vi "Grid_Finish_v1.vi"(8 "Error in":errorcluster, 9 "FileRefs":T2, 10 "Settings":T1={"Drift Correction Settings"={"Drift Correction every"=80, "Drift correction Pixels"=256, "Channel index (0-23)"=0, "MaxImagesBack"=2, "Threshold"=2, "Increment"=8, "max applied Drift Correction"=20, "Correct Drift"=TRUE, "Correlate"=0, "Correct z drift"=FALSE, "zdrift \nDuration (s)"=0.0}, "Spectroscopy Setting"={"Imaging Current"=1e-11, "ref Current"=7e-11, "tip Speed (m/s)"=2e-09, "Imaging Bias"=0.02, "ref Bias"=-0.1, "preSTS delay [ms]"=500, "STS z offset"=2e-10, "during Spec Bias (V)"=-0.1, "trigger1 < Hz"=0.0, "trigger 2 >Hz"=0.0, "autoStop"=FALSE, "Spectroscopy"=0, "PLL ON/OFF"=TRUE, "readjust setpoint every "=1, "z Reference"=FALSE, "Lock In"=TRUE}, "Misc"={"File name"="symmetric_node_zOff=200p", "Email when finished"="cornelius.krull@monash.edu,Dhaneesh.Gopalakrishnan@monash.edu,marina.castelli@monash.edu"}, "Grid Settings"={"type"=1, "type order"=1, "X pixel"=0, "Y pixel"=0, "Grid_Parms"={"center X (m)"=0.0, "center Y (m)"=0.0, "width (m)"=0.0, "height (m)"=0.0, "angle (deg)"=0.0}}} {"Grid Settings"."type order" items=["Grid", "Random", "Adam7"]; "Grid Settings"."type" items=["Line", "Grid"]; "Spectroscopy Setting"."Spectroscopy" items=["Bias", "zSpec"]; "Spectroscopy Setting"."trigger 2 >Hz" format="%#_6p"; "Spectroscopy Setting"."trigger1 < Hz" format="%#_6p"; "Spectroscopy Setting"."during Spec Bias (V)" format="%#_5p"; "Spectroscopy Setting"."STS z offset" format="%#_6p"; "Spectroscopy Setting"."ref Bias" format="%#_6p"; "Spectroscopy Setting"."Imaging Bias" format="%#_6p"; "Spectroscopy Setting"."tip Speed (m/s)" format="%.2p"; "Spectroscopy Setting"."ref Current" format="%#_6p"; "Spectroscopy Setting"."Imaging Current" format="%#_6p"; "Drift Correction Settings"."Correlate" items=["first Frame", "successive Frames"]; "Drift Correction Settings"."max applied Drift Correction" min=1 max=100 step=1 format="%.0p"; "Drift Correction Settings"."Threshold" min=1 step=1; "Drift Correction Settings"."Channel index (0-23)" items=["Current"=0, "Z (m)"=14]}, 11 "Application reference":refnum<vi>) -> ()   [LabVIEW 2014]
uses:
  <userlib>/Nanonis Prog Interface V5/Nanonis Prog Interface.lvlib
panel:
  # "z Spectroscopy"
  # "GRID points"
  # "Increase this if no Drift was detected for \na certain number of images"
  # "% of image size"
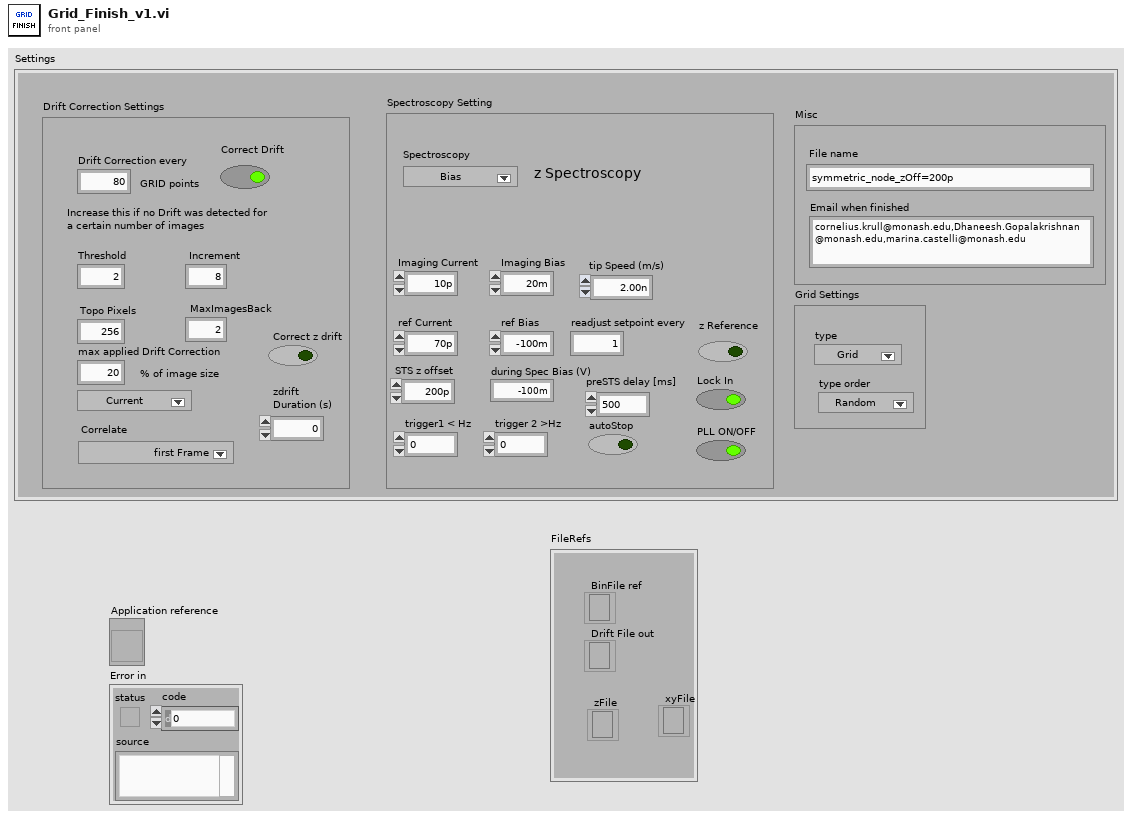
[diagram p1: front panel]
types:
  T1 = cluster{"Drift Correction Settings":cluster{"Drift Correction every":i32, "Drift correction Pixels":i32, "Channel index (0-23)":u8, "MaxImagesBack":i32, "Threshold":i32, "Increment":i32, "max applied Drift Correction":i32, "Correct Drift":bool, "Correlate":u16, "Correct z drift":bool, "zdrift \nDuration (s)":dbl}, "Spectroscopy Setting":cluster{"Imaging Current":dbl, "ref Current":dbl, "tip Speed (m/s)":sgl, "Imaging Bias":dbl, "ref Bias":dbl, "preSTS delay [ms]":u32, "STS z offset":dbl, "during Spec Bias (V)":sgl, "trigger1 < Hz":sgl, "trigger 2 >Hz":sgl, "autoStop":bool, "Spectroscopy":u16, "PLL ON/OFF":bool, "readjust setpoint every ":i32, "z Reference":bool, "Lock In":bool}, "Misc":cluster{"File name":string, "Email when finished":string}, "Grid Settings":cluster{"type":u16, "type order":u16, "X pixel":i32, "Y pixel":i32, "Grid_Parms":cluster{"center X (m)":sgl, "center Y (m)":sgl, "width (m)":sgl, "height (m)":sgl, "angle (deg)":sgl}}}
  T2 = cluster{"Drift File out":refnum<file>, "zFile":refnum<file>, "BinFile ref":refnum<file>, "xyFile":refnum<file>}
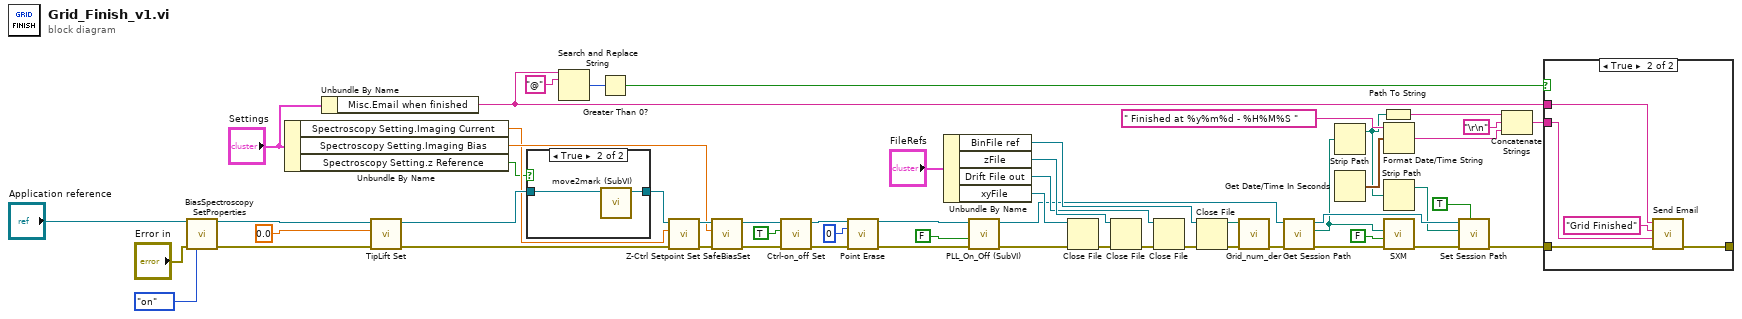
[diagram p0: block diagram]
diagram:
  n1 = call <userlib>:"BiasSpectroscopy SetProperties.vi"("Application ref in"="Application reference", "Error in (no error)"="Error in", "Z-Controller hold (no change)"=enum16{"no change", "on", "off"}."on") -> ("Application ref out"=w45:refnum<vi>, "Error out"=w14:errorcluster)  [unwired: 11 in]
  n2 = Unbundle By Name("Settings") -> ("Spectroscopy Setting.Imaging Current"=w10:dbl, "Spectroscopy Setting.Imaging Bias"=w11:dbl, "Spectroscopy Setting.z Reference"=w1:bool)
  n3 = Unbundle By Name("Settings") -> ("Misc.Email when finished"=w27:string)
  n4 = call <userlib>:"TipLift Set.vi"("error in (no error)"=w14, "TipLift (m)"=sgl 0.0, "Application ref in"=w45) -> ("error out"=w13:errorcluster, "Application ref out"=w42:refnum<vi>)  [unwired: 7 in]
  n5 = case shown="True" w1 {
    tunnel: w42 -> [w57 w59]
    tunnel: [w57 w58] -> w33
    frame False {
    }
    frame True {
      n6 = call "move2mark (SubVI).vi"("Application in"=w59) -> ("Application out"=w58:refnum<vi>)  [unwired: 10 in]
    }
  }
  n7 = Search and Replace String(input string=w27, search string="@") -> (number of replacements=w48:i32)  [unwired: 6 in, 3 out]
  n8 = Greater Than 0?(x=w48) -> (x > 0?=w47:bool)
  n9 = call <userlib>:"Z-Ctrl Setpoint Set.vi"("error in (no error)"=w13, "Z Controller setpoint"=w10, "Application ref in"=w33) -> ("error out"=w12:errorcluster, "Application ref out"=w32:refnum<vi>)  [unwired: 7 in]
  n10 = call "SafeBiasSet.vi"("Application ref in"=w32, "Bias (V)"=w11, "error in (no error)"=w12) -> ("Application ref out"=w39:refnum<vi>, "Error out"=w36:errorcluster)  [unwired: 6 in]
  n11 = call <userlib>:"Ctrl-on_off Set.vi"("error in (no error)"=w36, "Z Controller ON/OFF"=TRUE, "Application ref in"=w39) -> ("error out"=w35:errorcluster, "Application ref out"=w41:refnum<vi>)  [unwired: 7 in]
  n12 = call <userlib>:"Point Erase.vi"("Application ref in"=w41, "Point index (-1=All points)"=0, "error in (no error)"=w35) -> ("Application ref out"=w38:refnum<vi>, "error out"=w34:errorcluster)  [unwired: 11 in]
  n13 = Unbundle By Name("FileRefs") -> ("BinFile ref"=w19:refnum<file>, "zFile"=w25:refnum<file>, "Drift File out"=w23:refnum<file>, "xyFile"=w8:refnum<file>)
  n14 = call "PLL_On_Off (SubVI).vi"("error in (no error)"=w34, "Output ON/OFF (F=OFF)"=FALSE, "Application in"=w38) -> ("error out"=w2:errorcluster, "Application out"=w4:refnum<vi>)  [unwired: 7 in]
  n15 = Close File(refnum=w8, error in=w2) -> (error out=w7:errorcluster)  [unwired: 1 out]
  n16 = Close File(refnum=w25, error in=w7) -> (error out=w24:errorcluster)  [unwired: 1 out]
  n17 = Close File(refnum=w23, error in=w24) -> (error out=w21:errorcluster)  [unwired: 1 out]
  n18 = Close File(refnum=w19, error in=w21) -> (path=w22:path, error out=w20:errorcluster)
  n19 = call "Grid_num_der.vi"("error in (no error)"=w20, "Binary Spectroscopy File"=w22) -> ("error out"=w18:errorcluster)  [unwired: 9 in]
  n20 = call <userlib>:"Get Session Path.vi"("error in (no error)"=w18, "Application ref in"=w4) -> ("error out"=w55:errorcluster, "Session path"=w17:path, "Application ref out"=w29:refnum<vi>)  [unwired: 7 in]
  n21 = Strip Path(path=w17) -> (stripped path=w9:path)  [unwired: 1 out]
  n22 = Get Date/Time In Seconds() -> (seconds since 1Jan1904=w28:timestamp)
  n23 = Path To String(path=w9) -> (string=w54:string)
  n24 = Format Date/Time String(time format string (%c)=" Finished at %y%m%d - %H%M%S ", seconds (now)=w28) -> (date/time string=w51:string)  [unwired: 1 in]
  n25 = Strip Path(path=w9) -> (stripped path=w16:path)  [unwired: 1 out]
  n26 = call "SXM.vi"("Path"=w17, "Delete"=FALSE, "error in"=w55) -> ("error out"=w30:errorcluster)  [unwired: 7 in]
  n27 = call <userlib>:"Set Session Path.vi"("Save settings to previous? (False)"=TRUE, "error in (no error)"=w30, "Session Folder"=w16, "Application ref in"=w29) -> ("error out"=w15:errorcluster)  [unwired: 6 in, 1 out]
  n28 = Concatenate Strings(w54, "\r\n", w51) -> (w53:string)
  n29 = case shown="True" w47 {
    tunnel: w15 -> [w60 w65]
    tunnel: w53 -> [_ w63]
    tunnel: w27 -> [_ w62]
    tunnel: [w60 w61] -> _
    frame False {
    }
    frame True {
      n30 = call "Send Email"("error in"=w65, "Message"=w63, "Subject"="Grid Finished", "Recipients"=w62) -> ("error out"=w61:errorcluster)  [unwired: 7 in]
    }
  }
